vi "Plot.vi"(8 "error in (no error)":errorcluster, 11 "Data in":refnum<class "Data.lvclass">) -> (0 "error out":errorcluster, 3 "Data out":refnum<class "Data.lvclass">)   [LabVIEW 2015, in "MDSplus.lvlib" / "Data.lvclass"]
doc: "Plots the data in a newly created Scope instance."
uses:
  Data.lvclass
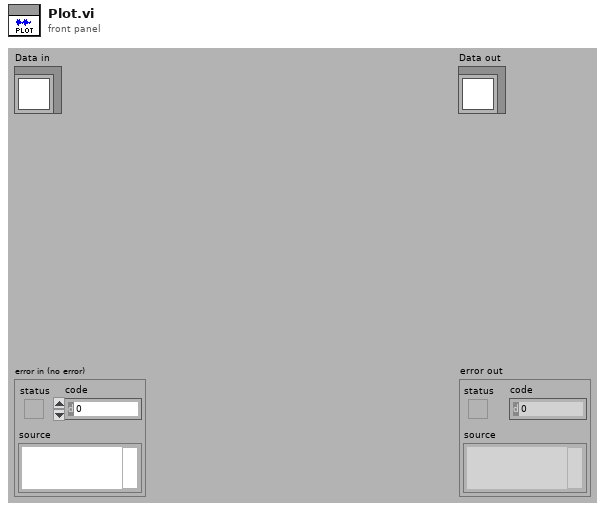
[diagram p1: front panel]
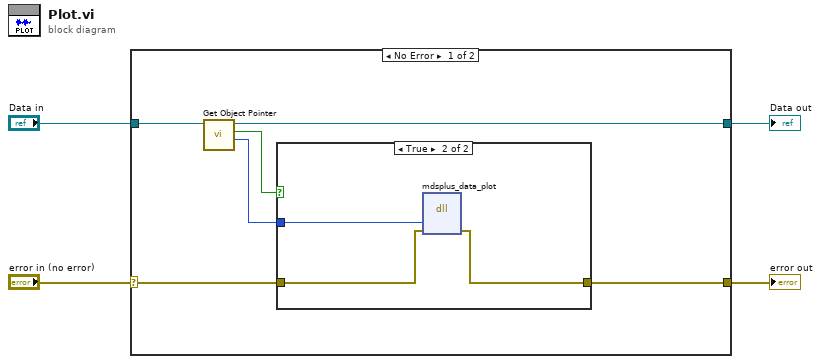
[diagram p0: block diagram]
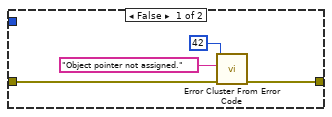
[diagram p2: hidden frame]
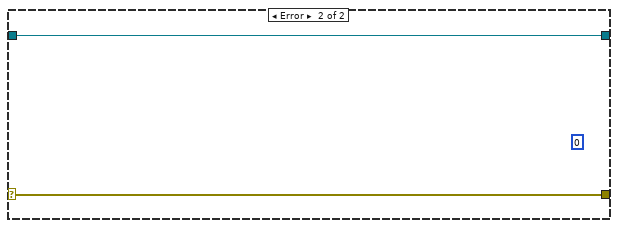
[diagram p3: hidden frame]
diagram:
  n1 = case shown="No Error" "error in (no error)" {
    selector: "error in (no error)" -> [w7 w19]
    tunnel: [w6 w19] -> w3
    tunnel: [w5 w18] -> w1
    tunnel: "Data in" -> [w10 w18]
    frame No Error {
      n2 = call-dynamic "Get Object Pointer.vi"("Data in"=w10) -> ("Object Pointer"=w8:i64, "Assigned object pointer?"=w9:bool, "Data out"=w5:refnum<class "Data.lvclass">)  [unwired: 8 in]
      n3 = case shown="True" w9 {
        tunnel: w8 -> [_ w17]
        tunnel: w7 -> [w12 w16]
        tunnel: [w11 w15] -> w6
        frame False {
          n4 = call <vilib>:"Error Cluster From Error Code.vi"("error in (no error)"=w12, "error message (\"\")"="Object pointer not assigned." ("error message (\"\")"), "error code (0)"=42) -> ("error out"=w11:errorcluster)  [unwired: 6 in]
        }
        frame True {
          n5 = dll-call lib="MDSobjectsLVShr" fn="mdsplus_data_plot"("lvDataPtr"=w17, "error"=w16) -> ("error"=w15:errorcluster)  [unwired: 5 in, 2 out]
        }
      }
    }
    frame Error {
      (unwired) i8 0 ("floatOut")
    }
  }
  "error out" <- w3
  "Data out" <- w1
